vi "deserialize (Frames).vi"(11 "data in":string[][](array[string])) -> (3 "frames":map{string, T1}(c390))   [LabVIEW 2020]
uses:
  _controls/1553_Frames.ctl
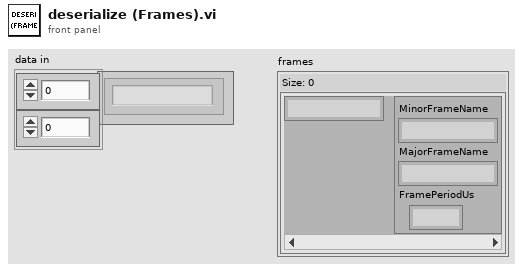
[diagram p1: front panel]
types:
  T1 = typedef "1553_Frames.ctl" = cluster{"MinorFrameName":string, "MajorFrameName":string, "FramePeriodUs":i32}
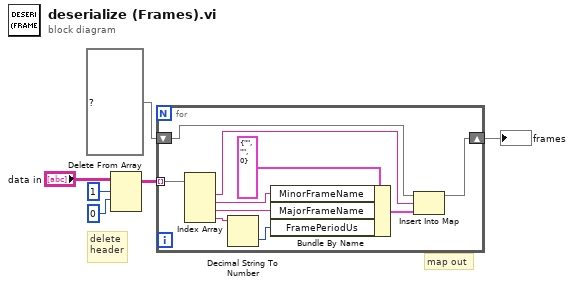
[diagram p0: block diagram]
diagram:
  # "delete\nheader"
  # "map out"
  n1 = Delete From Array(array="data in", length=1, index (row)=0) -> (array with subset deleted=w2:string[][])  [unwired: 1 in, 1 out]
  n2 = for {
    tunnel: w2 -> [w16] mode=indexing
    shift-right: [w14] -> w6
    shift-left: map{string, T1} {} ("map") -> [w15]
    n3 = Index Array(array=w16) -> (element #1=w10:string, element #2=w13:string, element #3=w11:string, element #4=w9:string)  [unwired: 4 in]
    n4 = Decimal String To Number(string=w9) -> (number=w8:i32)  [unwired: 2 in, 1 out]
    n5 = Bundle By Name(cluster=T1 {"MinorFrameName"="", "MajorFrameName"="", "FramePeriodUs"=0} ("frames"), "MinorFrameName"=w13, "MajorFrameName"=w11, "FramePeriodUs"=w8) -> (w7:T1)
    n6 = Insert Into Map(map in=w15, key=w10, value=w7) -> (map out=w14:map{string, T1})  [unwired: 2 out]
  }
  "frames" <- w6
